vi "Initialize.vi"(5 "Password":string, 7 "Username":string, 8 "error in (no error)":errorcluster, 10 "Address":string, 11 "WebDAV in":refnum<class "WebDAV.lvclass">) -> (0 "error out":errorcluster, 3 "WebDAV out":refnum<class "WebDAV.lvclass">)   [LabVIEW 2015, in "RT Management.lvlib" / "WebDAV.lvclass"]
uses:
  WebDAV.lvclass
  File Transfer Behavior/File Transfer Behavior.lvclass/File Transfer Behavior.ctl
  WebDAV.lvclass/WebDAV.ctl
  File Transfer Behavior/Set Username.vi
  File Transfer Behavior/Set Password.vi
  File Transfer Behavior/Set Address.vi
  File Transfer Behavior/Get Password.vi
  File Transfer Behavior/Get Username.vi
  File Transfer Behavior/Get Address.vi
  Set Session.vi
  <vilib>/WebDAVClient/NI_WebDAV.lvlib
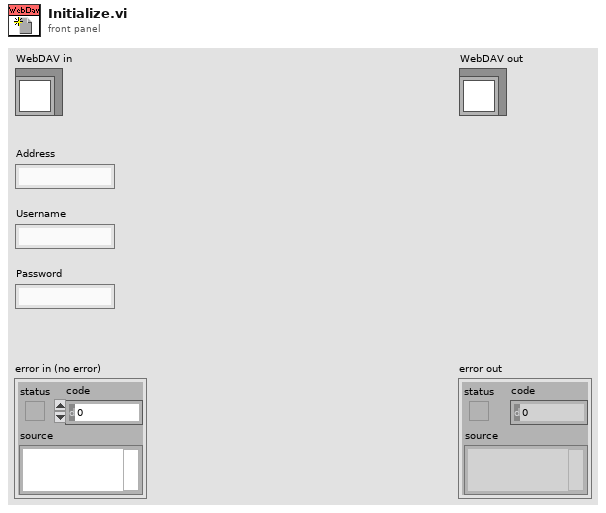
[diagram p1: front panel]
types:
  T1 = typedef "NI_WebDAV.lvlib/SessionHandle.ctl" = refnum<k1>
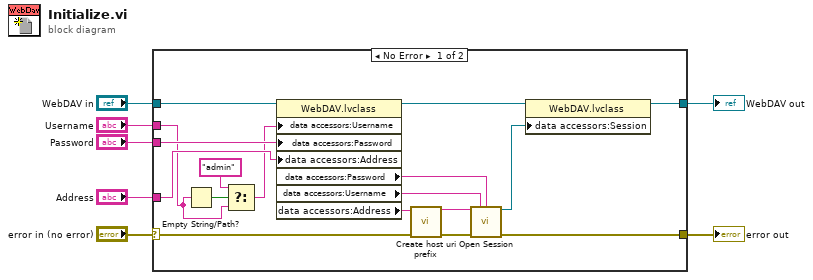
[diagram p0: block diagram]
diagram:
  n1 = case shown="No Error" "error in (no error)" {
    selector: "error in (no error)" -> [w18 w25]
    tunnel: "WebDAV in" -> [w16 w26]
    tunnel: [w20 w25] -> w7
    tunnel: [w19 w26] -> w6
    tunnel: "Address" -> [w10 _]
    tunnel: "Username" -> [w9 _]
    tunnel: "Password" -> [w13 _]
    frame No Error {
      n2 = Empty String/Path?(string/path=w9) -> (empty?=w12:bool)
      n3 = Select(t="admin", s=w12, f=w9) -> (s? t:f=w8:string)
      n4 = property class="WebDAV.lvclass"(reference=w16, "data accessors:Username"=w8, "data accessors:Password"=w13, "data accessors:Address"=w10) -> (reference out=w15:refnum<class "WebDAV.lvclass">, "data accessors:Password"=w14:string, "data accessors:Username"=w21:string, "data accessors:Address"=w24:string)  [unwired: 1 in, 1 out]
      n5 = call "Create host uri prefix.vi"("error in (no error)"=w18, "address"=w24) -> ("error out"=w23:errorcluster, "host uri prefix"=w22:string)  [unwired: 8 in]
      n6 = call <vilib>:"Open Session.vi"("host uri prefix"=w22, "username"=w21, "password"=w14, "error in (no error)"=w23) -> ("session handle out"=w17:T1, "error out"=w20:errorcluster)  [unwired: 10 in]
      n7 = property class="WebDAV.lvclass"(reference=w15, "data accessors:Session"=w17) -> (reference out=w19:refnum<class "WebDAV.lvclass">)  [unwired: 1 in, 1 out]
    }
    frame Error {
    }
  }
  "error out" <- w7
  "WebDAV out" <- w6
